vi "Autonomous Independent.vi"() -> ()   [LabVIEW 2020]
doc: "This VI is called when autonomous begins, and will automatically be terminated when autonomous ends. You can carry out timed or sensor driven robot movement independently without needing to return to the caller."
uses:
  <vilib>/Rock Robotics/WPI/DriverStation/WPI_DriverStationAllianceInfo.ctl
  <vilib>/Rock Robotics/Network Tables/NT Read String.vi
  Robot Global Data.vi
panel:
  out "Alliance":T1
  out "Front Left Drive Position":dbl
  out "Navx  Comp Yaw":dbl
  out "Auto Step":dbl
  # "Be sure to right-click and choose Data Operations>>Make Current Value default if you want to save the array values with the VI"
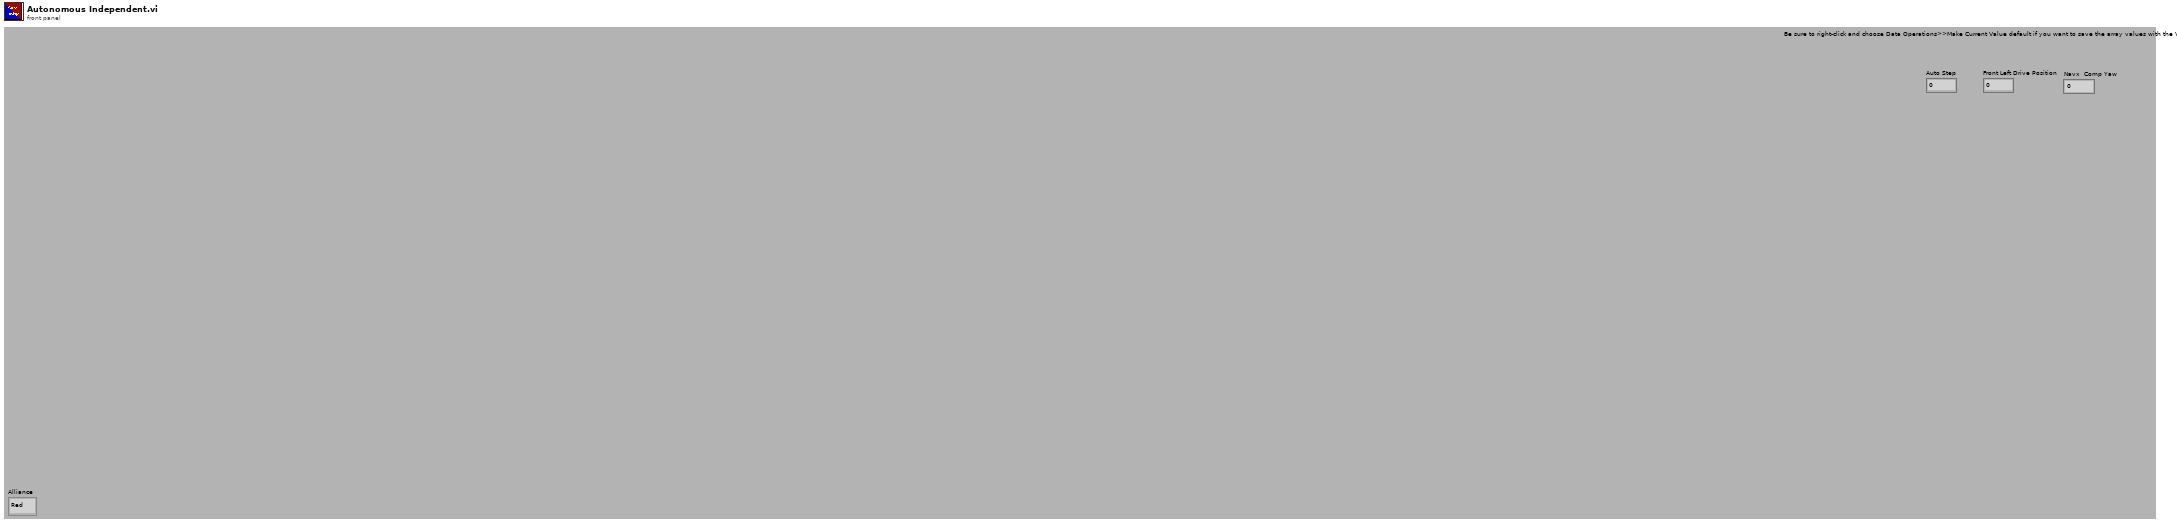
[diagram p1: front panel]
types:
  T1 = typedef "WPI_DriverStationAllianceInfo.ctl" = enum16{"Red", "Blue", "Invalid"}
  T2 = typedef "Direction Commands.ctl" = cluster{"Lateral - X":dbl, "Longitudinal - Y":dbl, "Rotational - Z":dbl}
  T3 = typedef "Drive Comands.ctl" = cluster{"Align Steer Motors":bool, "Brake":bool, "Coast":bool, "Autonomous":bool}
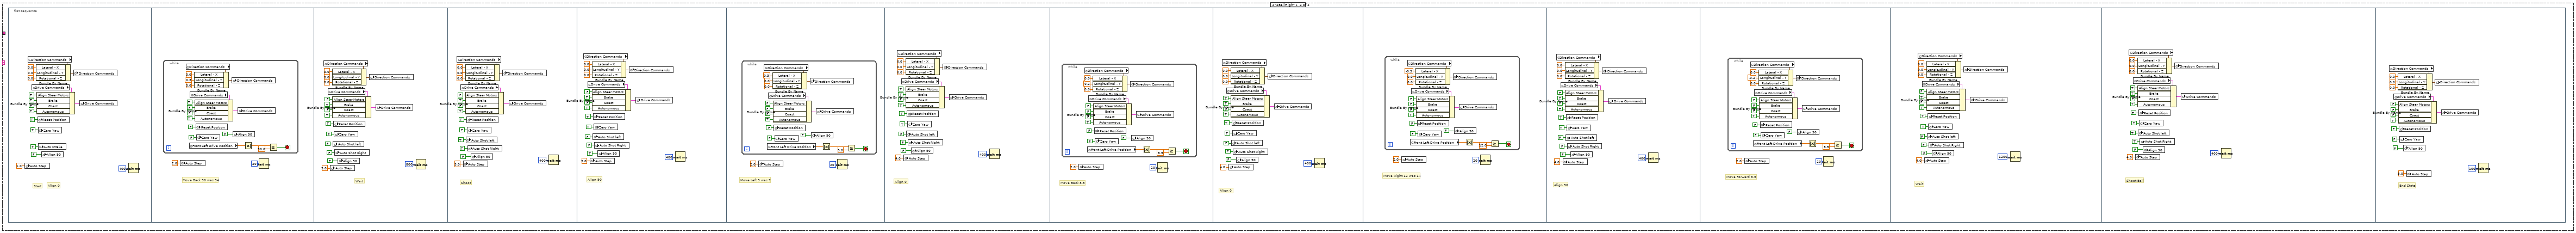
[diagram p2: hidden frame]
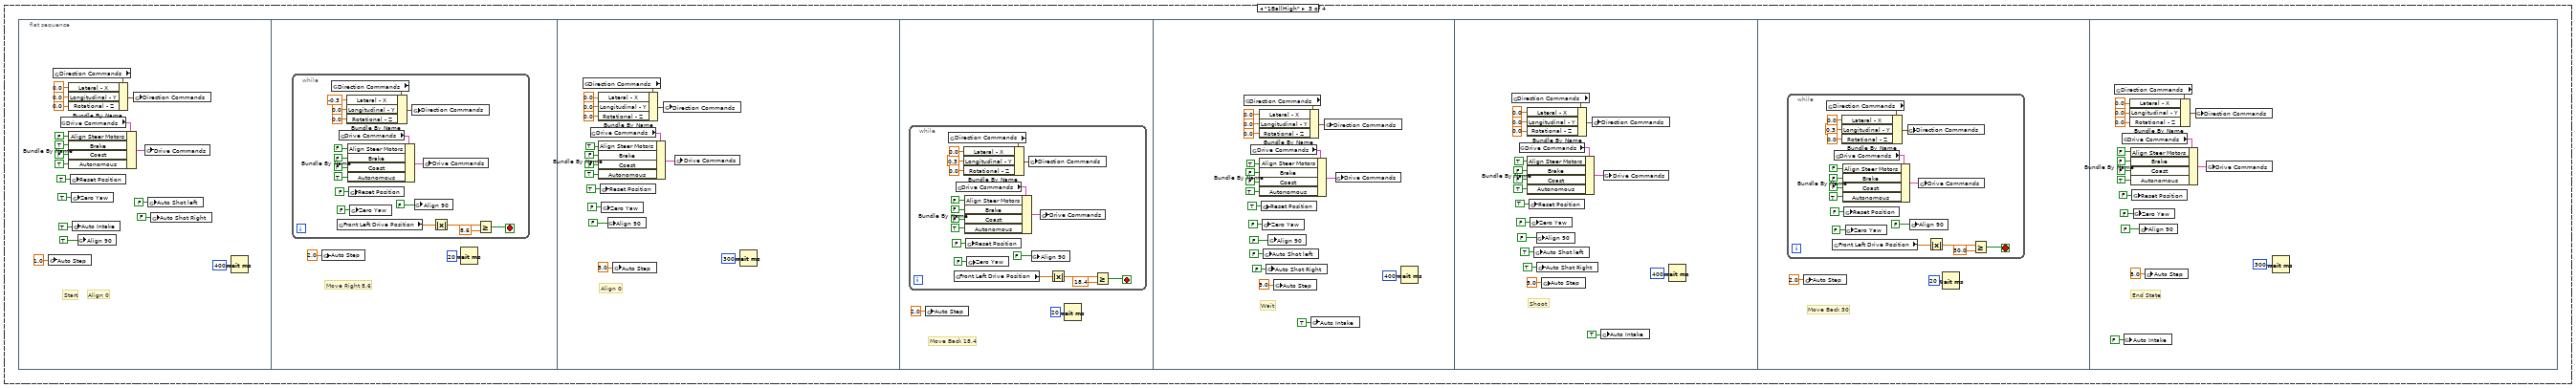
[diagram p3: hidden frame]
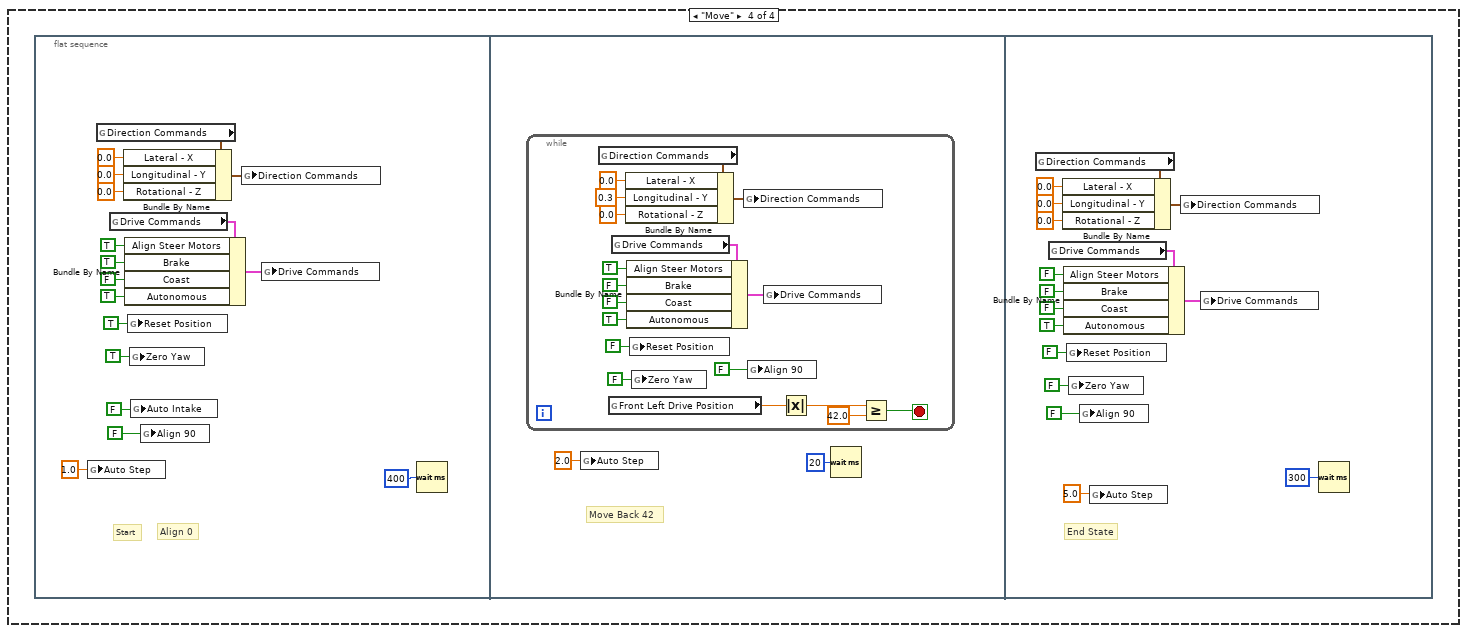
[diagram p4: hidden frame]
diagram:
  (unwired) "This function is run in parallel when the autonomous period begins. It will be terminated automatically when the period ends.\n\nNote that all Driver Station inputs are automatically latched and will not change once auto begins."
  # "Back Long + value\nForward Long - Value\nRight  - Value\nLeft + Value"
  # "The game specific data sent by FMS"
  # "This tells you the autonomous selected in the \ndashboard. Begin.vi publishes the Auto List values\nby writing a constant to the dashboard.\nUpdate the constant to add or modify the name\nof an autonomous."
  # "Every 20ms, report that we are running autonomous\ncode. Loop will abort the same time as the VI."
  # "This tells you the driver position\nand alliance color"
  n1 = call <vilib>:"WPI_DriverStationGet Alliance Info.vi"() -> ("Alliance"=w6:T1)  [unwired: 6 in, 5 out]
  "Alliance" <- w6
  n2 = call <vilib>:"WPI_DriverStationGame Specific Data.vi"() -> ("Game Specific Data"=w7:string)  [unwired: 11 in]
  n3 = while {
    stop <- FALSE stop-if-true
    n4 = call <vilib>:"WPI_DriverStationReport Robot Code State.vi"("Autonomous"=TRUE) -> ()  [unwired: 10 in, 1 out]
    n5 = Wait (ms)(milliseconds to wait=u32 20) -> ()  [unwired: 1 out]
  }
  n6 = Equal?(x=w6, y=WPI_DriverStationAllianceInfo."Red") -> (x = y?=w4:bool)
  n7 = call-poly <vilib>:"NT Read Value.vi"("Name"="Auto Selector") -> ("String"=w8:string)  [unwired: 9 in, 1 out]
  n8 = Select(t="Red" ("Right Color Match 2"), s=w4, f="Blue" ("Right Color Match 2")) -> (s? t:f=w1:string)
  n9 = global write "Robot Global Data.vi" "Alliance Color"(w1) -> ()
  n10 = case shown="\"3Ball\", Default" w8 {
    tunnel: w7 -> [_ _ _ _]
    frame "3Ball", Default {
      n11 = flat-sequence {
        frame #0 {
          # "Align 0"
          # "Start"
          n12 = global write "Robot Global Data.vi" "Auto Step"(1.0 ("Auto Step")) -> ()
          n13 = global read "Robot Global Data.vi" "Direction Commands"() -> (w23:T2)
          n14 = global read "Robot Global Data.vi" "Drive Commands"() -> (w22:T3)
          n15 = Bundle By Name(cluster=w23, "Lateral - X"=0.0, "Longitudinal - Y"=0.0, "Rotational - Z"=0.0) -> (w29:T2)
          n16 = Bundle By Name(cluster=w22, "Align Steer Motors"=TRUE, "Brake"=TRUE, "Coast"=FALSE, "Autonomous"=TRUE) -> (w21:T3)
          n17 = global write "Robot Global Data.vi" "Reset Position"(TRUE ("Reset Position")) -> ()
          n18 = global write "Robot Global Data.vi" "Zero Yaw"(TRUE ("Zero Yaw")) -> ()
          n19 = global write "Robot Global Data.vi" "Auto Intake"(TRUE ("Auto Intake")) -> ()
          n20 = global write "Robot Global Data.vi" "Align 90"(FALSE ("Auto Intake")) -> ()
          n21 = global write "Robot Global Data.vi" "Direction Commands"(w29) -> ()
          n22 = global write "Robot Global Data.vi" "Drive Commands"(w21) -> ()
          n23 = Wait (ms)(milliseconds to wait=u32 400) -> ()  [unwired: 1 out]
        }
        frame #1 {
          # "Move Back 32"
          n24 = while {
            stop <- w34 stop-if-true
            n25 = global read "Robot Global Data.vi" "Direction Commands"() -> (w43:T2)
            n26 = global read "Robot Global Data.vi" "Front Left Drive Position"() -> (w36:dbl)
            n27 = global read "Robot Global Data.vi" "Drive Commands"() -> (w42:T3)
            n28 = Bundle By Name(cluster=w43, "Lateral - X"=0.0, "Longitudinal - Y"=0.3, "Rotational - Z"=0.0) -> (w49:T2)
            n29 = Bundle By Name(cluster=w42, "Align Steer Motors"=TRUE, "Brake"=FALSE, "Coast"=FALSE, "Autonomous"=TRUE) -> (w41:T3)
            n30 = global write "Robot Global Data.vi" "Reset Position"(FALSE ("Reset Position")) -> ()
            n31 = global write "Robot Global Data.vi" "Zero Yaw"(FALSE ("Zero Yaw")) -> ()
            n32 = global write "Robot Global Data.vi" "Direction Commands"(w49) -> ()
            n33 = global write "Robot Global Data.vi" "Align 90"(FALSE ("Auto Intake")) -> ()
            n34 = global write "Robot Global Data.vi" "Drive Commands"(w41) -> ()
            n35 = Absolute Value(x=w36) -> (abs(x)=w33:dbl)
            n36 = Greater Or Equal?(x=w33, y=32.0) -> (x >= y?=w34:bool)
          }
          n37 = global write "Robot Global Data.vi" "Auto Step"(2.0 ("Auto Step")) -> ()
          n38 = Wait (ms)(milliseconds to wait=u32 20) -> ()  [unwired: 1 out]
        }
        frame #2 {
          # "Align 90 Stop"
          n39 = global read "Robot Global Data.vi" "Direction Commands"() -> (w61:T2)
          n40 = global read "Robot Global Data.vi" "Drive Commands"() -> (w60:T3)
          n41 = global write "Robot Global Data.vi" "Auto Step"(3.0 ("Auto Step")) -> ()
          n42 = Bundle By Name(cluster=w61, "Lateral - X"=0.0, "Longitudinal - Y"=0.0, "Rotational - Z"=0.0) -> (w67:T2)
          n43 = Bundle By Name(cluster=w60, "Align Steer Motors"=TRUE, "Brake"=TRUE, "Coast"=FALSE, "Autonomous"=TRUE) -> (w59:T3)
          n44 = global write "Robot Global Data.vi" "Auto Shot left"(FALSE ("Auto Shot left")) -> ()
          n45 = global write "Robot Global Data.vi" "Reset Position"(TRUE ("Reset Position")) -> ()
          n46 = global write "Robot Global Data.vi" "Zero Yaw"(TRUE ("Zero Yaw")) -> ()
          n47 = global write "Robot Global Data.vi" "Auto Shot Right"(FALSE ("Auto Shot Right")) -> ()
          n48 = global write "Robot Global Data.vi" "Align 90"(TRUE ("Auto Intake")) -> ()
          n49 = global write "Robot Global Data.vi" "Direction Commands"(w67) -> ()
          n50 = global write "Robot Global Data.vi" "Drive Commands"(w59) -> ()
          n51 = Wait (ms)(milliseconds to wait=u32 400) -> ()  [unwired: 1 out]
        }
        frame #3 {
          # "Shoot"
          n52 = global read "Robot Global Data.vi" "Direction Commands"() -> (w79:T2)
          n53 = global read "Robot Global Data.vi" "Drive Commands"() -> (w78:T3)
          n54 = global write "Robot Global Data.vi" "Auto Step"(3.0 ("Auto Step")) -> ()
          n55 = Bundle By Name(cluster=w79, "Lateral - X"=0.0, "Longitudinal - Y"=0.0, "Rotational - Z"=0.0) -> (w85:T2)
          n56 = Bundle By Name(cluster=w78, "Align Steer Motors"=TRUE, "Brake"=TRUE, "Coast"=FALSE, "Autonomous"=TRUE) -> (w77:T3)
          n57 = global write "Robot Global Data.vi" "Auto Shot left"(TRUE ("Auto Shot left")) -> ()
          n58 = global write "Robot Global Data.vi" "Reset Position"(TRUE ("Reset Position")) -> ()
          n59 = global write "Robot Global Data.vi" "Zero Yaw"(TRUE ("Zero Yaw")) -> ()
          n60 = global write "Robot Global Data.vi" "Auto Shot Right"(TRUE ("Auto Shot Right")) -> ()
          n61 = global write "Robot Global Data.vi" "Align 90"(TRUE ("Auto Intake")) -> ()
          n62 = global write "Robot Global Data.vi" "Direction Commands"(w85) -> ()
          n63 = global write "Robot Global Data.vi" "Drive Commands"(w77) -> ()
          n64 = Wait (ms)(milliseconds to wait=u32 400) -> ()  [unwired: 1 out]
        }
        frame #4 {
          # "Move Right 6"
          n65 = while {
            stop <- w90 stop-if-true
            n66 = global read "Robot Global Data.vi" "Direction Commands"() -> (w99:T2)
            n67 = global read "Robot Global Data.vi" "Front Left Drive Position"() -> (w92:dbl)
            n68 = global read "Robot Global Data.vi" "Drive Commands"() -> (w98:T3)
            n69 = Bundle By Name(cluster=w99, "Lateral - X"=-0.2, "Longitudinal - Y"=0.0, "Rotational - Z"=0.0) -> (w105:T2)
            n70 = Bundle By Name(cluster=w98, "Align Steer Motors"=FALSE, "Brake"=FALSE, "Coast"=FALSE, "Autonomous"=TRUE) -> (w97:T3)
            n71 = global write "Robot Global Data.vi" "Reset Position"(FALSE ("Reset Position")) -> ()
            n72 = global write "Robot Global Data.vi" "Zero Yaw"(FALSE ("Zero Yaw")) -> ()
            n73 = global write "Robot Global Data.vi" "Direction Commands"(w105) -> ()
            n74 = global write "Robot Global Data.vi" "Align 90"(FALSE ("Auto Intake")) -> ()
            n75 = global write "Robot Global Data.vi" "Drive Commands"(w97) -> ()
            n76 = Absolute Value(x=w92) -> (abs(x)=w89:dbl)
            n77 = Greater Or Equal?(x=w89, y=6.0) -> (x >= y?=w90:bool)
          }
          n78 = global write "Robot Global Data.vi" "Auto Step"(2.0 ("Auto Step")) -> ()
          n79 = Wait (ms)(milliseconds to wait=u32 20) -> ()  [unwired: 1 out]
        }
        frame #5 {
          # "Align 0"
          n80 = global read "Robot Global Data.vi" "Direction Commands"() -> (w117:T2)
          n81 = global read "Robot Global Data.vi" "Drive Commands"() -> (w116:T3)
          n82 = global write "Robot Global Data.vi" "Auto Step"(3.0 ("Auto Step")) -> ()
          n83 = Bundle By Name(cluster=w117, "Lateral - X"=0.0, "Longitudinal - Y"=0.0, "Rotational - Z"=0.0) -> (w123:T2)
          n84 = Bundle By Name(cluster=w116, "Align Steer Motors"=TRUE, "Brake"=TRUE, "Coast"=FALSE, "Autonomous"=TRUE) -> (w115:T3)
          n85 = global write "Robot Global Data.vi" "Auto Shot left"(FALSE ("Auto Shot left")) -> ()
          n86 = global write "Robot Global Data.vi" "Reset Position"(TRUE ("Reset Position")) -> ()
          n87 = global write "Robot Global Data.vi" "Zero Yaw"(TRUE ("Zero Yaw")) -> ()
          n88 = global write "Robot Global Data.vi" "Auto Shot Right"(FALSE ("Auto Shot Right")) -> ()
          n89 = global write "Robot Global Data.vi" "Align 90"(FALSE ("Auto Intake")) -> ()
          n90 = global write "Robot Global Data.vi" "Direction Commands"(w123) -> ()
          n91 = global write "Robot Global Data.vi" "Drive Commands"(w115) -> ()
          n92 = Wait (ms)(milliseconds to wait=u32 400) -> ()  [unwired: 1 out]
        }
        frame #6 {
          # "Move Back 9 was 12"
          n93 = while {
            stop <- w128 stop-if-true
            n94 = global read "Robot Global Data.vi" "Direction Commands"() -> (w137:T2)
            n95 = global read "Robot Global Data.vi" "Front Left Drive Position"() -> (w130:dbl)
            n96 = global read "Robot Global Data.vi" "Drive Commands"() -> (w136:T3)
            n97 = Bundle By Name(cluster=w137, "Lateral - X"=0.0, "Longitudinal - Y"=0.2, "Rotational - Z"=0.0) -> (w143:T2)
            n98 = Bundle By Name(cluster=w136, "Align Steer Motors"=FALSE, "Brake"=FALSE, "Coast"=FALSE, "Autonomous"=TRUE) -> (w135:T3)
            n99 = global write "Robot Global Data.vi" "Reset Position"(FALSE ("Reset Position")) -> ()
            n100 = global write "Robot Global Data.vi" "Zero Yaw"(FALSE ("Zero Yaw")) -> ()
            n101 = global write "Robot Global Data.vi" "Direction Commands"(w143) -> ()
            n102 = global write "Robot Global Data.vi" "Align 90"(FALSE ("Auto Intake")) -> ()
            n103 = global write "Robot Global Data.vi" "Drive Commands"(w135) -> ()
            n104 = Absolute Value(x=w130) -> (abs(x)=w127:dbl)
            n105 = Greater Or Equal?(x=w127, y=9.0) -> (x >= y?=w128:bool)
          }
          n106 = global write "Robot Global Data.vi" "Auto Step"(4.0 ("Auto Step")) -> ()
          n107 = Wait (ms)(milliseconds to wait=u32 20) -> ()  [unwired: 1 out]
        }
        frame #7 {
          # "Align 0"
          n108 = global read "Robot Global Data.vi" "Direction Commands"() -> (w155:T2)
          n109 = global read "Robot Global Data.vi" "Drive Commands"() -> (w154:T3)
          n110 = global write "Robot Global Data.vi" "Auto Step"(5.0 ("Auto Step")) -> ()
          n111 = Bundle By Name(cluster=w155, "Lateral - X"=0.0, "Longitudinal - Y"=0.0, "Rotational - Z"=0.0) -> (w161:T2)
          n112 = Bundle By Name(cluster=w154, "Align Steer Motors"=TRUE, "Brake"=TRUE, "Coast"=FALSE, "Autonomous"=TRUE) -> (w153:T3)
          n113 = global write "Robot Global Data.vi" "Auto Shot left"(FALSE ("Auto Shot left")) -> ()
          n114 = global write "Robot Global Data.vi" "Reset Position"(TRUE ("Reset Position")) -> ()
          n115 = global write "Robot Global Data.vi" "Zero Yaw"(TRUE ("Zero Yaw")) -> ()
          n116 = global write "Robot Global Data.vi" "Auto Shot Right"(FALSE ("Auto Shot Right")) -> ()
          n117 = global write "Robot Global Data.vi" "Direction Commands"(w161) -> ()
          n118 = global write "Robot Global Data.vi" "Drive Commands"(w153) -> ()
          n119 = global write "Robot Global Data.vi" "Align 90"(FALSE ("Auto Intake")) -> ()
          n120 = Wait (ms)(milliseconds to wait=u32 400) -> ()  [unwired: 1 out]
        }
        frame #8 {
          # "Move Forward 30 was 32"
          n121 = while {
            stop <- w166 stop-if-true
            n122 = global read "Robot Global Data.vi" "Direction Commands"() -> (w175:T2)
            n123 = global read "Robot Global Data.vi" "Front Left Drive Position"() -> (w168:dbl)
            n124 = global read "Robot Global Data.vi" "Drive Commands"() -> (w174:T3)
            n125 = Bundle By Name(cluster=w175, "Lateral - X"=0.0, "Longitudinal - Y"=-0.3, "Rotational - Z"=0.0) -> (w181:T2)
            n126 = Bundle By Name(cluster=w174, "Align Steer Motors"=FALSE, "Brake"=FALSE, "Coast"=FALSE, "Autonomous"=TRUE) -> (w173:T3)
            n127 = global write "Robot Global Data.vi" "Reset Position"(FALSE ("Reset Position")) -> ()
            n128 = global write "Robot Global Data.vi" "Zero Yaw"(FALSE ("Zero Yaw")) -> ()
            n129 = global write "Robot Global Data.vi" "Direction Commands"(w181) -> ()
            n130 = global write "Robot Global Data.vi" "Drive Commands"(w173) -> ()
            n131 = Absolute Value(x=w168) -> (abs(x)=w165:dbl)
            n132 = global write "Robot Global Data.vi" "Align 90"(FALSE ("Auto Intake")) -> ()
            n133 = Greater Or Equal?(x=w165, y=30.0) -> (x >= y?=w166:bool)
          }
          n134 = global write "Robot Global Data.vi" "Auto Step"(6.0 ("Auto Step")) -> ()
          n135 = Wait (ms)(milliseconds to wait=u32 20) -> ()  [unwired: 1 out]
        }
        frame #9 {
          # "Align 90"
          n136 = global read "Robot Global Data.vi" "Direction Commands"() -> (w193:T2)
          n137 = global read "Robot Global Data.vi" "Drive Commands"() -> (w192:T3)
          n138 = Bundle By Name(cluster=w193, "Lateral - X"=0.0, "Longitudinal - Y"=0.0, "Rotational - Z"=0.0) -> (w199:T2)
          n139 = Bundle By Name(cluster=w192, "Align Steer Motors"=FALSE, "Brake"=TRUE, "Coast"=FALSE, "Autonomous"=TRUE) -> (w191:T3)
          n140 = global write "Robot Global Data.vi" "Reset Position"(TRUE ("Reset Position")) -> ()
          n141 = global write "Robot Global Data.vi" "Auto Shot left"(FALSE ("Auto Shot left")) -> ()
          n142 = global write "Robot Global Data.vi" "Zero Yaw"(TRUE ("Zero Yaw")) -> ()
          n143 = global write "Robot Global Data.vi" "Auto Shot Right"(FALSE ("Auto Shot Right")) -> ()
          n144 = global write "Robot Global Data.vi" "Auto Step"(7.0 ("Auto Step")) -> ()
          n145 = global write "Robot Global Data.vi" "Direction Commands"(w199) -> ()
          n146 = global write "Robot Global Data.vi" "Drive Commands"(w191) -> ()
          n147 = global write "Robot Global Data.vi" "Align 90"(TRUE ("Auto Intake")) -> ()
          n148 = Wait (ms)(milliseconds to wait=u32 400) -> ()  [unwired: 1 out]
        }
        frame #10 {
          # "Move Left 57 was 51"
          n149 = while {
            stop <- w204 stop-if-true
            n150 = global read "Robot Global Data.vi" "Direction Commands"() -> (w213:T2)
            n151 = global read "Robot Global Data.vi" "Front Left Drive Position"() -> (w206:dbl)
            n152 = global read "Robot Global Data.vi" "Drive Commands"() -> (w212:T3)
            n153 = Bundle By Name(cluster=w213, "Lateral - X"=0.3, "Longitudinal - Y"=0.0, "Rotational - Z"=0.0) -> (w219:T2)
            n154 = Bundle By Name(cluster=w212, "Align Steer Motors"=FALSE, "Brake"=FALSE, "Coast"=FALSE, "Autonomous"=TRUE) -> (w211:T3)
            n155 = global write "Robot Global Data.vi" "Reset Position"(FALSE ("Reset Position")) -> ()
            n156 = global write "Robot Global Data.vi" "Zero Yaw"(FALSE ("Zero Yaw")) -> ()
            n157 = global write "Robot Global Data.vi" "Direction Commands"(w219) -> ()
            n158 = global write "Robot Global Data.vi" "Drive Commands"(w211) -> ()
            n159 = Absolute Value(x=w206) -> (abs(x)=w203:dbl)
            n160 = global write "Robot Global Data.vi" "Align 90"(FALSE ("Auto Intake")) -> ()
            n161 = Greater Or Equal?(x=w203, y=57.0) -> (x >= y?=w204:bool)
          }
          n162 = global write "Robot Global Data.vi" "Auto Step"(8.0 ("Auto Step")) -> ()
          n163 = Wait (ms)(milliseconds to wait=u32 20) -> ()  [unwired: 1 out]
        }
        frame #11 {
          # "Aign 0"
          n164 = global read "Robot Global Data.vi" "Direction Commands"() -> (w231:T2)
          n165 = global read "Robot Global Data.vi" "Drive Commands"() -> (w230:T3)
          n166 = global write "Robot Global Data.vi" "Auto Step"(5.0 ("Auto Step")) -> ()
          n167 = Bundle By Name(cluster=w231, "Lateral - X"=0.0, "Longitudinal - Y"=0.0, "Rotational - Z"=0.0) -> (w237:T2)
          n168 = Bundle By Name(cluster=w230, "Align Steer Motors"=TRUE, "Brake"=TRUE, "Coast"=FALSE, "Autonomous"=TRUE) -> (w229:T3)
          n169 = global write "Robot Global Data.vi" "Auto Shot left"(FALSE ("Auto Shot left")) -> ()
          n170 = global write "Robot Global Data.vi" "Reset Position"(TRUE ("Reset Position")) -> ()
          n171 = global write "Robot Global Data.vi" "Zero Yaw"(TRUE ("Zero Yaw")) -> ()
          n172 = global write "Robot Global Data.vi" "Auto Shot Right"(FALSE ("Auto Shot Right")) -> ()
          n173 = global write "Robot Global Data.vi" "Direction Commands"(w237) -> ()
          n174 = global write "Robot Global Data.vi" "Drive Commands"(w229) -> ()
          n175 = global write "Robot Global Data.vi" "Align 90"(FALSE ("Auto Intake")) -> ()
          n176 = Wait (ms)(milliseconds to wait=u32 400) -> ()  [unwired: 1 out]
        }
        frame #12 {
          # "Move Back 12 was 19"
          n177 = while {
            stop <- w242 stop-if-true
            n178 = global read "Robot Global Data.vi" "Direction Commands"() -> (w251:T2)
            n179 = global read "Robot Global Data.vi" "Front Left Drive Position"() -> (w244:dbl)
            n180 = global read "Robot Global Data.vi" "Drive Commands"() -> (w250:T3)
            n181 = Bundle By Name(cluster=w251, "Lateral - X"=0.0, "Longitudinal - Y"=0.3, "Rotational - Z"=0.0) -> (w257:T2)
            n182 = Bundle By Name(cluster=w250, "Align Steer Motors"=FALSE, "Brake"=FALSE, "Coast"=FALSE, "Autonomous"=TRUE) -> (w249:T3)
            n183 = global write "Robot Global Data.vi" "Reset Position"(FALSE ("Reset Position")) -> ()
            n184 = global write "Robot Global Data.vi" "Zero Yaw"(FALSE ("Zero Yaw")) -> ()
            n185 = global write "Robot Global Data.vi" "Direction Commands"(w257) -> ()
            n186 = global write "Robot Global Data.vi" "Drive Commands"(w249) -> ()
            n187 = Absolute Value(x=w244) -> (abs(x)=w241:dbl)
            n188 = global write "Robot Global Data.vi" "Align 90"(FALSE ("Auto Intake")) -> ()
            n189 = Greater Or Equal?(x=w241, y=12.0) -> (x >= y?=w242:bool)
          }
          n190 = global write "Robot Global Data.vi" "Auto Step"(6.0 ("Auto Step")) -> ()
          n191 = Wait (ms)(milliseconds to wait=u32 20) -> ()  [unwired: 1 out]
        }
        frame #13 {
          # "Align 90"
          n192 = global read "Robot Global Data.vi" "Direction Commands"() -> (w269:T2)
          n193 = global read "Robot Global Data.vi" "Drive Commands"() -> (w268:T3)
          n194 = Bundle By Name(cluster=w269, "Lateral - X"=0.0, "Longitudinal - Y"=0.0, "Rotational - Z"=0.0) -> (w275:T2)
          n195 = Bundle By Name(cluster=w268, "Align Steer Motors"=FALSE, "Brake"=TRUE, "Coast"=FALSE, "Autonomous"=TRUE) -> (w267:T3)
          n196 = global write "Robot Global Data.vi" "Reset Position"(TRUE ("Reset Position")) -> ()
          n197 = global write "Robot Global Data.vi" "Auto Shot left"(FALSE ("Auto Shot left")) -> ()
          n198 = global write "Robot Global Data.vi" "Zero Yaw"(TRUE ("Zero Yaw")) -> ()
          n199 = global write "Robot Global Data.vi" "Auto Shot Right"(FALSE ("Auto Shot Right")) -> ()
          n200 = global write "Robot Global Data.vi" "Auto Step"(7.0 ("Auto Step")) -> ()
          n201 = global write "Robot Global Data.vi" "Direction Commands"(w275) -> ()
          n202 = global write "Robot Global Data.vi" "Drive Commands"(w267) -> ()
          n203 = global write "Robot Global Data.vi" "Align 90"(TRUE ("Auto Intake")) -> ()
          n204 = Wait (ms)(milliseconds to wait=u32 400) -> ()  [unwired: 1 out]
        }
        frame #14 {
          # "Move Right  45 was 48 was 39"
          n205 = while {
            stop <- w280 stop-if-true
            n206 = global read "Robot Global Data.vi" "Direction Commands"() -> (w289:T2)
            n207 = global read "Robot Global Data.vi" "Front Left Drive Position"() -> (w282:dbl)
            n208 = global read "Robot Global Data.vi" "Drive Commands"() -> (w288:T3)
            n209 = Bundle By Name(cluster=w289, "Lateral - X"=-0.3, "Longitudinal - Y"=0.0, "Rotational - Z"=0.0) -> (w295:T2)
            n210 = Bundle By Name(cluster=w288, "Align Steer Motors"=FALSE, "Brake"=FALSE, "Coast"=FALSE, "Autonomous"=TRUE) -> (w287:T3)
            n211 = global write "Robot Global Data.vi" "Reset Position"(FALSE ("Reset Position")) -> ()
            n212 = global write "Robot Global Data.vi" "Zero Yaw"(FALSE ("Zero Yaw")) -> ()
            n213 = global write "Robot Global Data.vi" "Direction Commands"(w295) -> ()
            n214 = global write "Robot Global Data.vi" "Drive Commands"(w287) -> ()
            n215 = Absolute Value(x=w282) -> (abs(x)=w279:dbl)
            n216 = global write "Robot Global Data.vi" "Align 90"(FALSE ("Auto Intake")) -> ()
            n217 = Greater Or Equal?(x=w279, y=45.0) -> (x >= y?=w280:bool)
          }
          n218 = global write "Robot Global Data.vi" "Auto Step"(8.0 ("Auto Step")) -> ()
          n219 = Wait (ms)(milliseconds to wait=u32 20) -> ()  [unwired: 1 out]
        }
        frame #15 {
          # "Align 0"
          n220 = global read "Robot Global Data.vi" "Direction Commands"() -> (w305:T2)
          n221 = global read "Robot Global Data.vi" "Drive Commands"() -> (w306:T3)
          n222 = global write "Robot Global Data.vi" "Auto Shot left"(FALSE ("Auto Shot left")) -> ()
          n223 = global write "Robot Global Data.vi" "Auto Shot Right"(FALSE ("Auto Shot Right")) -> ()
          n224 = Bundle By Name(cluster=w305, "Lateral - X"=0.0, "Longitudinal - Y"=0.0, "Rotational - Z"=0.0) -> (w299:T2)
          n225 = Bundle By Name(cluster=w306, "Align Steer Motors"=TRUE, "Brake"=TRUE, "Coast"=FALSE, "Autonomous"=TRUE) -> (w307:T3)
          n226 = global write "Robot Global Data.vi" "Reset Position"(TRUE ("Reset Position")) -> ()
          n227 = global write "Robot Global Data.vi" "Zero Yaw"(TRUE ("Zero Yaw")) -> ()
          n228 = global write "Robot Global Data.vi" "Auto Step"(9.0 ("Auto Step")) -> ()
          n229 = global write "Robot Global Data.vi" "Direction Commands"(w299) -> ()
          n230 = global write "Robot Global Data.vi" "Drive Commands"(w307) -> ()
          n231 = global write "Robot Global Data.vi" "Align 90"(FALSE ("Auto Intake")) -> ()
          n232 = Wait (ms)(milliseconds to wait=u32 400) -> ()  [unwired: 1 out]
        }
        frame #16 {
          # "Wait"
          n233 = global read "Robot Global Data.vi" "Direction Commands"() -> (w325:T2)
          n234 = global read "Robot Global Data.vi" "Drive Commands"() -> (w324:T3)
          n235 = global write "Robot Global Data.vi" "Auto Step"(4.0 ("Auto Step")) -> ()
          n236 = Bundle By Name(cluster=w325, "Lateral - X"=0.0, "Longitudinal - Y"=0.0, "Rotational - Z"=0.0) -> (w331:T2)
          n237 = Bundle By Name(cluster=w324, "Align Steer Motors"=FALSE, "Brake"=TRUE, "Coast"=FALSE, "Autonomous"=TRUE) -> (w323:T3)
          n238 = global write "Robot Global Data.vi" "Auto Shot left"(FALSE ("Auto Shot left")) -> ()
          n239 = global write "Robot Global Data.vi" "Reset Position"(TRUE ("Reset Position")) -> ()
          n240 = global write "Robot Global Data.vi" "Zero Yaw"(TRUE ("Zero Yaw")) -> ()
          n241 = global write "Robot Global Data.vi" "Auto Shot Right"(FALSE ("Auto Shot Right")) -> ()
          n242 = global write "Robot Global Data.vi" "Align 90"(FALSE ("Auto Intake")) -> ()
          n243 = global write "Robot Global Data.vi" "Direction Commands"(w331) -> ()
          n244 = global write "Robot Global Data.vi" "Drive Commands"(w323) -> ()
          n245 = Wait (ms)(milliseconds to wait=u32 800) -> ()  [unwired: 1 out]
        }
        frame #17 {
          # "Align 0"
          n246 = global read "Robot Global Data.vi" "Direction Commands"() -> (w341:T2)
          n247 = global read "Robot Global Data.vi" "Drive Commands"() -> (w342:T3)
          n248 = global write "Robot Global Data.vi" "Auto Shot left"(FALSE ("Auto Shot left")) -> ()
          n249 = global write "Robot Global Data.vi" "Auto Shot Right"(FALSE ("Auto Shot Right")) -> ()
          n250 = Bundle By Name(cluster=w341, "Lateral - X"=0.0, "Longitudinal - Y"=0.0, "Rotational - Z"=0.0) -> (w335:T2)
          n251 = Bundle By Name(cluster=w342, "Align Steer Motors"=TRUE, "Brake"=TRUE, "Coast"=FALSE, "Autonomous"=TRUE) -> (w343:T3)
          n252 = global write "Robot Global Data.vi" "Reset Position"(TRUE ("Reset Position")) -> ()
          n253 = global write "Robot Global Data.vi" "Zero Yaw"(TRUE ("Zero Yaw")) -> ()
          n254 = global write "Robot Global Data.vi" "Auto Step"(9.0 ("Auto Step")) -> ()
          n255 = global write "Robot Global Data.vi" "Direction Commands"(w335) -> ()
          n256 = global write "Robot Global Data.vi" "Drive Commands"(w343) -> ()
          n257 = global write "Robot Global Data.vi" "Align 90"(FALSE ("Auto Intake")) -> ()
          n258 = Wait (ms)(milliseconds to wait=u32 400) -> ()  [unwired: 1 out]
        }
        frame #18 {
          # "Align 0 and Shoot"
          n259 = global read "Robot Global Data.vi" "Direction Commands"() -> (w359:T2)
          n260 = global read "Robot Global Data.vi" "Drive Commands"() -> (w360:T3)
          n261 = Bundle By Name(cluster=w359, "Lateral - X"=0.0, "Longitudinal - Y"=0.0, "Rotational - Z"=0.0) -> (w353:T2)
          n262 = Bundle By Name(cluster=w360, "Align Steer Motors"=TRUE, "Brake"=TRUE, "Coast"=FALSE, "Autonomous"=TRUE) -> (w361:T3)
          n263 = global write "Robot Global Data.vi" "Reset Position"(TRUE ("Reset Position")) -> ()
          n264 = global write "Robot Global Data.vi" "Zero Yaw"(TRUE ("Zero Yaw")) -> ()
          n265 = global write "Robot Global Data.vi" "Align 90"(FALSE ("Auto Intake")) -> ()
          n266 = global write "Robot Global Data.vi" "Auto Step"(11.0 ("Auto Step")) -> ()
          n267 = global write "Robot Global Data.vi" "Direction Commands"(w353) -> ()
          n268 = global write "Robot Global Data.vi" "Drive Commands"(w361) -> ()
          n269 = global write "Robot Global Data.vi" "Auto Shot left"(TRUE ("Auto Shot left")) -> ()
          n270 = global write "Robot Global Data.vi" "Auto Shot Right"(FALSE ("Auto Shot Right")) -> ()
          n271 = Wait (ms)(milliseconds to wait=u32 200) -> ()  [unwired: 1 out]
        }
        frame #19 {
          # "Align 0 and Shoot"
          n272 = global read "Robot Global Data.vi" "Direction Commands"() -> (w377:T2)
          n273 = global read "Robot Global Data.vi" "Drive Commands"() -> (w378:T3)
          n274 = Bundle By Name(cluster=w377, "Lateral - X"=0.0, "Longitudinal - Y"=0.0, "Rotational - Z"=0.0) -> (w371:T2)
          n275 = Bundle By Name(cluster=w378, "Align Steer Motors"=TRUE, "Brake"=TRUE, "Coast"=FALSE, "Autonomous"=TRUE) -> (w379:T3)
          n276 = global write "Robot Global Data.vi" "Reset Position"(TRUE ("Reset Position")) -> ()
          n277 = global write "Robot Global Data.vi" "Zero Yaw"(TRUE ("Zero Yaw")) -> ()
          n278 = global write "Robot Global Data.vi" "Align 90"(FALSE ("Auto Intake")) -> ()
          n279 = global write "Robot Global Data.vi" "Auto Step"(11.0 ("Auto Step")) -> ()
          n280 = global write "Robot Global Data.vi" "Direction Commands"(w371) -> ()
          n281 = global write "Robot Global Data.vi" "Drive Commands"(w379) -> ()
          n282 = global write "Robot Global Data.vi" "Auto Shot left"(FALSE ("Auto Shot left")) -> ()
          n283 = global write "Robot Global Data.vi" "Auto Shot Right"(TRUE ("Auto Shot Right")) -> ()
          n284 = Wait (ms)(milliseconds to wait=u32 200) -> ()  [unwired: 1 out]
        }
        frame #20 {
          # "End State"
          n285 = global read "Robot Global Data.vi" "Direction Commands"() -> (w395:T2)
          n286 = global read "Robot Global Data.vi" "Drive Commands"() -> (w394:T3)
          n287 = Bundle By Name(cluster=w395, "Lateral - X"=0.0, "Longitudinal - Y"=0.0, "Rotational - Z"=0.0) -> (w401:T2)
          n288 = Bundle By Name(cluster=w394, "Align Steer Motors"=FALSE, "Brake"=FALSE, "Coast"=FALSE, "Autonomous"=TRUE) -> (w393:T3)
          n289 = global write "Robot Global Data.vi" "Reset Position"(FALSE ("Reset Position")) -> ()
          n290 = global write "Robot Global Data.vi" "Zero Yaw"(FALSE ("Zero Yaw")) -> ()
          n291 = global write "Robot Global Data.vi" "Align 90"(FALSE ("Auto Intake")) -> ()
          n292 = global write "Robot Global Data.vi" "Auto Step"(18.0 ("Auto Step")) -> ()
          n293 = global write "Robot Global Data.vi" "Direction Commands"(w401) -> ()
          n294 = global write "Robot Global Data.vi" "Drive Commands"(w393) -> ()
          n295 = Wait (ms)(milliseconds to wait=u32 300) -> ()  [unwired: 1 out]
        }
      }
    }
    frame "2BallHigh" {
      n296 = flat-sequence {
        frame #0 {
          # "Align 0"
          # "Start"
          n297 = global write "Robot Global Data.vi" "Auto Step"(1.0 ("Auto Step")) -> ()
          n298 = global read "Robot Global Data.vi" "Direction Commands"() -> (w412:T2)
          n299 = global read "Robot Global Data.vi" "Drive Commands"() -> (w411:T3)
          n300 = Bundle By Name(cluster=w412, "Lateral - X"=0.0, "Longitudinal - Y"=0.0, "Rotational - Z"=0.0) -> (w418:T2)
          n301 = Bundle By Name(cluster=w411, "Align Steer Motors"=TRUE, "Brake"=TRUE, "Coast"=FALSE, "Autonomous"=TRUE) -> (w410:T3)
          n302 = global write "Robot Global Data.vi" "Reset Position"(TRUE ("Reset Position")) -> ()
          n303 = global write "Robot Global Data.vi" "Zero Yaw"(TRUE ("Zero Yaw")) -> ()
          n304 = global write "Robot Global Data.vi" "Auto Intake"(TRUE ("Auto Intake")) -> ()
          n305 = global write "Robot Global Data.vi" "Align 90"(FALSE ("Auto Intake")) -> ()
          n306 = global write "Robot Global Data.vi" "Direction Commands"(w418) -> ()
          n307 = global write "Robot Global Data.vi" "Drive Commands"(w410) -> ()
          n308 = Wait (ms)(milliseconds to wait=u32 400) -> ()  [unwired: 1 out]
        }
        frame #1 {
          # "Move Back 30 was 34"
          n309 = while {
            stop <- w423 stop-if-true
            n310 = global read "Robot Global Data.vi" "Direction Commands"() -> (w432:T2)
            n311 = global read "Robot Global Data.vi" "Front Left Drive Position"() -> (w425:dbl)
            n312 = global read "Robot Global Data.vi" "Drive Commands"() -> (w431:T3)
            n313 = Bundle By Name(cluster=w432, "Lateral - X"=0.0, "Longitudinal - Y"=0.3, "Rotational - Z"=0.0) -> (w438:T2)
            n314 = Bundle By Name(cluster=w431, "Align Steer Motors"=TRUE, "Brake"=FALSE, "Coast"=FALSE, "Autonomous"=TRUE) -> (w430:T3)
            n315 = global write "Robot Global Data.vi" "Reset Position"(FALSE ("Reset Position")) -> ()
            n316 = global write "Robot Global Data.vi" "Zero Yaw"(FALSE ("Zero Yaw")) -> ()
            n317 = global write "Robot Global Data.vi" "Direction Commands"(w438) -> ()
            n318 = global write "Robot Global Data.vi" "Align 90"(FALSE ("Auto Intake")) -> ()
            n319 = global write "Robot Global Data.vi" "Drive Commands"(w430) -> ()
            n320 = Absolute Value(x=w425) -> (abs(x)=w422:dbl)
            n321 = Greater Or Equal?(x=w422, y=30.0) -> (x >= y?=w423:bool)
          }
          n322 = global write "Robot Global Data.vi" "Auto Step"(2.0 ("Auto Step")) -> ()
          n323 = Wait (ms)(milliseconds to wait=u32 20) -> ()  [unwired: 1 out]
        }
        frame #2 {
          # "Wait"
          n324 = global read "Robot Global Data.vi" "Direction Commands"() -> (w450:T2)
          n325 = global read "Robot Global Data.vi" "Drive Commands"() -> (w449:T3)
          n326 = global write "Robot Global Data.vi" "Auto Step"(3.0 ("Auto Step")) -> ()
          n327 = Bundle By Name(cluster=w450, "Lateral - X"=0.0, "Longitudinal - Y"=0.0, "Rotational - Z"=0.0) -> (w456:T2)
          n328 = Bundle By Name(cluster=w449, "Align Steer Motors"=FALSE, "Brake"=TRUE, "Coast"=FALSE, "Autonomous"=TRUE) -> (w448:T3)
          n329 = global write "Robot Global Data.vi" "Auto Shot left"(FALSE ("Auto Shot left")) -> ()
          n330 = global write "Robot Global Data.vi" "Reset Position"(TRUE ("Reset Position")) -> ()
          n331 = global write "Robot Global Data.vi" "Zero Yaw"(FALSE ("Zero Yaw")) -> ()
          n332 = global write "Robot Global Data.vi" "Auto Shot Right"(FALSE ("Auto Shot Right")) -> ()
          n333 = global write "Robot Global Data.vi" "Align 90"(FALSE ("Auto Intake")) -> ()
          n334 = global write "Robot Global Data.vi" "Direction Commands"(w456) -> ()
          n335 = global write "Robot Global Data.vi" "Drive Commands"(w448) -> ()
          n336 = Wait (ms)(milliseconds to wait=u32 800) -> ()  [unwired: 1 out]
        }
        frame #3 {
          # "Shoot"
          n337 = global read "Robot Global Data.vi" "Direction Commands"() -> (w468:T2)
          n338 = global read "Robot Global Data.vi" "Drive Commands"() -> (w467:T3)
          n339 = global write "Robot Global Data.vi" "Auto Step"(3.0 ("Auto Step")) -> ()
          n340 = Bundle By Name(cluster=w468, "Lateral - X"=0.0, "Longitudinal - Y"=0.0, "Rotational - Z"=0.0) -> (w474:T2)
          n341 = Bundle By Name(cluster=w467, "Align Steer Motors"=FALSE, "Brake"=TRUE, "Coast"=FALSE, "Autonomous"=TRUE) -> (w466:T3)
          n342 = global write "Robot Global Data.vi" "Auto Shot left"(TRUE ("Auto Shot left")) -> ()
          n343 = global write "Robot Global Data.vi" "Reset Position"(TRUE ("Reset Position")) -> ()
          n344 = global write "Robot Global Data.vi" "Zero Yaw"(FALSE ("Zero Yaw")) -> ()
          n345 = global write "Robot Global Data.vi" "Auto Shot Right"(TRUE ("Auto Shot Right")) -> ()
          n346 = global write "Robot Global Data.vi" "Align 90"(FALSE ("Auto Intake")) -> ()
          n347 = global write "Robot Global Data.vi" "Direction Commands"(w474) -> ()
          n348 = global write "Robot Global Data.vi" "Drive Commands"(w466) -> ()
          n349 = Wait (ms)(milliseconds to wait=u32 400) -> ()  [unwired: 1 out]
        }
        frame #4 {
          # "Align 90"
          n350 = global read "Robot Global Data.vi" "Direction Commands"() -> (w486:T2)
          n351 = global read "Robot Global Data.vi" "Drive Commands"() -> (w485:T3)
          n352 = global write "Robot Global Data.vi" "Auto Step"(3.0 ("Auto Step")) -> ()
          n353 = Bundle By Name(cluster=w486, "Lateral - X"=0.0, "Longitudinal - Y"=0.0, "Rotational - Z"=0.0) -> (w492:T2)
          n354 = Bundle By Name(cluster=w485, "Align Steer Motors"=FALSE, "Brake"=TRUE, "Coast"=FALSE, "Autonomous"=TRUE) -> (w484:T3)
          n355 = global write "Robot Global Data.vi" "Auto Shot left"(FALSE ("Auto Shot left")) -> ()
          n356 = global write "Robot Global Data.vi" "Reset Position"(TRUE ("Reset Position")) -> ()
          n357 = global write "Robot Global Data.vi" "Zero Yaw"(TRUE ("Zero Yaw")) -> ()
          n358 = global write "Robot Global Data.vi" "Auto Shot Right"(FALSE ("Auto Shot Right")) -> ()
          n359 = global write "Robot Global Data.vi" "Align 90"(TRUE ("Auto Intake")) -> ()
          n360 = global write "Robot Global Data.vi" "Direction Commands"(w492) -> ()
          n361 = global write "Robot Global Data.vi" "Drive Commands"(w484) -> ()
          n362 = Wait (ms)(milliseconds to wait=u32 400) -> ()  [unwired: 1 out]
        }
        frame #5 {
          # "Move Left 5 was 7"
          n363 = while {
            stop <- w497 stop-if-true
            n364 = global read "Robot Global Data.vi" "Direction Commands"() -> (w506:T2)
            n365 = global read "Robot Global Data.vi" "Front Left Drive Position"() -> (w499:dbl)
            n366 = global read "Robot Global Data.vi" "Drive Commands"() -> (w505:T3)
            n367 = Bundle By Name(cluster=w506, "Lateral - X"=0.3, "Longitudinal - Y"=0.0, "Rotational - Z"=0.0) -> (w512:T2)
            n368 = Bundle By Name(cluster=w505, "Align Steer Motors"=FALSE, "Brake"=FALSE, "Coast"=FALSE, "Autonomous"=TRUE) -> (w504:T3)
            n369 = global write "Robot Global Data.vi" "Reset Position"(FALSE ("Reset Position")) -> ()
            n370 = global write "Robot Global Data.vi" "Zero Yaw"(FALSE ("Zero Yaw")) -> ()
            n371 = global write "Robot Global Data.vi" "Direction Commands"(w512) -> ()
            n372 = global write "Robot Global Data.vi" "Align 90"(FALSE ("Auto Intake")) -> ()
            n373 = global write "Robot Global Data.vi" "Drive Commands"(w504) -> ()
            n374 = Absolute Value(x=w499) -> (abs(x)=w496:dbl)
            n375 = Greater Or Equal?(x=w496, y=5.0) -> (x >= y?=w497:bool)
          }
          n376 = global write "Robot Global Data.vi" "Auto Step"(2.0 ("Auto Step")) -> ()
          n377 = Wait (ms)(milliseconds to wait=u32 20) -> ()  [unwired: 1 out]
        }
        frame #6 {
          # "Align 0"
          n378 = global read "Robot Global Data.vi" "Direction Commands"() -> (w524:T2)
          n379 = global read "Robot Global Data.vi" "Drive Commands"() -> (w523:T3)
          n380 = global write "Robot Global Data.vi" "Auto Step"(4.0 ("Auto Step")) -> ()
          n381 = Bundle By Name(cluster=w524, "Lateral - X"=0.0, "Longitudinal - Y"=0.0, "Rotational - Z"=0.0) -> (w530:T2)
          n382 = Bundle By Name(cluster=w523, "Align Steer Motors"=TRUE, "Brake"=TRUE, "Coast"=FALSE, "Autonomous"=TRUE) -> (w522:T3)
          n383 = global write "Robot Global Data.vi" "Auto Shot left"(FALSE ("Auto Shot left")) -> ()
          n384 = global write "Robot Global Data.vi" "Reset Position"(TRUE ("Reset Position")) -> ()
          n385 = global write "Robot Global Data.vi" "Zero Yaw"(TRUE ("Zero Yaw")) -> ()
          n386 = global write "Robot Global Data.vi" "Auto Shot Right"(FALSE ("Auto Shot Right")) -> ()
          n387 = global write "Robot Global Data.vi" "Align 90"(FALSE ("Auto Intake")) -> ()
          n388 = global write "Robot Global Data.vi" "Direction Commands"(w530) -> ()
          n389 = global write "Robot Global Data.vi" "Drive Commands"(w522) -> ()
          n390 = Wait (ms)(milliseconds to wait=u32 400) -> ()  [unwired: 1 out]
        }
        frame #7 {
          # "Move Back 8.5"
          n391 = while {
            stop <- w535 stop-if-true
            n392 = global read "Robot Global Data.vi" "Direction Commands"() -> (w544:T2)
            n393 = global read "Robot Global Data.vi" "Front Left Drive Position"() -> (w537:dbl)
            n394 = global read "Robot Global Data.vi" "Drive Commands"() -> (w543:T3)
            n395 = Bundle By Name(cluster=w544, "Lateral - X"=0.0, "Longitudinal - Y"=0.2, "Rotational - Z"=0.0) -> (w550:T2)
            n396 = Bundle By Name(cluster=w543, "Align Steer Motors"=FALSE, "Brake"=FALSE, "Coast"=FALSE, "Autonomous"=TRUE) -> (w542:T3)
            n397 = global write "Robot Global Data.vi" "Reset Position"(FALSE ("Reset Position")) -> ()
            n398 = global write "Robot Global Data.vi" "Zero Yaw"(FALSE ("Zero Yaw")) -> ()
            n399 = global write "Robot Global Data.vi" "Direction Commands"(w550) -> ()
            n400 = global write "Robot Global Data.vi" "Align 90"(FALSE ("Auto Intake")) -> ()
            n401 = global write "Robot Global Data.vi" "Drive Commands"(w542) -> ()
            n402 = Absolute Value(x=w537) -> (abs(x)=w534:dbl)
            n403 = Greater Or Equal?(x=w534, y=8.5) -> (x >= y?=w535:bool)
          }
          n404 = global write "Robot Global Data.vi" "Auto Step"(2.0 ("Auto Step")) -> ()
          n405 = Wait (ms)(milliseconds to wait=u32 20) -> ()  [unwired: 1 out]
        }
        frame #8 {
          # "Align 0"
          n406 = global read "Robot Global Data.vi" "Direction Commands"() -> (w562:T2)
          n407 = global read "Robot Global Data.vi" "Drive Commands"() -> (w561:T3)
          n408 = global write "Robot Global Data.vi" "Auto Step"(4.0 ("Auto Step")) -> ()
          n409 = Bundle By Name(cluster=w562, "Lateral - X"=0.0, "Longitudinal - Y"=0.0, "Rotational - Z"=0.0) -> (w568:T2)
          n410 = Bundle By Name(cluster=w561, "Align Steer Motors"=TRUE, "Brake"=TRUE, "Coast"=FALSE, "Autonomous"=TRUE) -> (w560:T3)
          n411 = global write "Robot Global Data.vi" "Auto Shot left"(FALSE ("Auto Shot left")) -> ()
          n412 = global write "Robot Global Data.vi" "Reset Position"(TRUE ("Reset Position")) -> ()
          n413 = global write "Robot Global Data.vi" "Zero Yaw"(TRUE ("Zero Yaw")) -> ()
          n414 = global write "Robot Global Data.vi" "Auto Shot Right"(FALSE ("Auto Shot Right")) -> ()
          n415 = global write "Robot Global Data.vi" "Align 90"(FALSE ("Auto Intake")) -> ()
          n416 = global write "Robot Global Data.vi" "Direction Commands"(w568) -> ()
          n417 = global write "Robot Global Data.vi" "Drive Commands"(w560) -> ()
          n418 = Wait (ms)(milliseconds to wait=u32 400) -> ()  [unwired: 1 out]
        }
        frame #9 {
          # "Move Right 12 was 14"
          n419 = while {
            stop <- w573 stop-if-true
            n420 = global read "Robot Global Data.vi" "Direction Commands"() -> (w582:T2)
            n421 = global read "Robot Global Data.vi" "Front Left Drive Position"() -> (w575:dbl)
            n422 = global read "Robot Global Data.vi" "Drive Commands"() -> (w581:T3)
            n423 = Bundle By Name(cluster=w582, "Lateral - X"=-0.3, "Longitudinal - Y"=0.0, "Rotational - Z"=0.0) -> (w588:T2)
            n424 = Bundle By Name(cluster=w581, "Align Steer Motors"=FALSE, "Brake"=FALSE, "Coast"=FALSE, "Autonomous"=TRUE) -> (w580:T3)
            n425 = global write "Robot Global Data.vi" "Reset Position"(FALSE ("Reset Position")) -> ()
            n426 = global write "Robot Global Data.vi" "Zero Yaw"(FALSE ("Zero Yaw")) -> ()
            n427 = global write "Robot Global Data.vi" "Direction Commands"(w588) -> ()
            n428 = global write "Robot Global Data.vi" "Align 90"(FALSE ("Auto Intake")) -> ()
            n429 = global write "Robot Global Data.vi" "Drive Commands"(w580) -> ()
            n430 = Absolute Value(x=w575) -> (abs(x)=w572:dbl)
            n431 = Greater Or Equal?(x=w572, y=12.0) -> (x >= y?=w573:bool)
          }
          n432 = global write "Robot Global Data.vi" "Auto Step"(2.0 ("Auto Step")) -> ()
          n433 = Wait (ms)(milliseconds to wait=u32 20) -> ()  [unwired: 1 out]
        }
        frame #10 {
          # "Align 90"
          n434 = global read "Robot Global Data.vi" "Direction Commands"() -> (w600:T2)
          n435 = global read "Robot Global Data.vi" "Drive Commands"() -> (w599:T3)
          n436 = global write "Robot Global Data.vi" "Auto Step"(4.0 ("Auto Step")) -> ()
          n437 = Bundle By Name(cluster=w600, "Lateral - X"=0.0, "Longitudinal - Y"=0.0, "Rotational - Z"=0.0) -> (w606:T2)
          n438 = Bundle By Name(cluster=w599, "Align Steer Motors"=FALSE, "Brake"=TRUE, "Coast"=FALSE, "Autonomous"=TRUE) -> (w598:T3)
          n439 = global write "Robot Global Data.vi" "Auto Shot left"(FALSE ("Auto Shot left")) -> ()
          n440 = global write "Robot Global Data.vi" "Reset Position"(TRUE ("Reset Position")) -> ()
          n441 = global write "Robot Global Data.vi" "Zero Yaw"(TRUE ("Zero Yaw")) -> ()
          n442 = global write "Robot Global Data.vi" "Auto Shot Right"(FALSE ("Auto Shot Right")) -> ()
          n443 = global write "Robot Global Data.vi" "Align 90"(FALSE ("Auto Intake")) -> ()
          n444 = global write "Robot Global Data.vi" "Direction Commands"(w606) -> ()
          n445 = global write "Robot Global Data.vi" "Drive Commands"(w598) -> ()
          n446 = Wait (ms)(milliseconds to wait=u32 400) -> ()  [unwired: 1 out]
        }
        frame #11 {
          # "Move Forward 8.5"
          n447 = while {
            stop <- w611 stop-if-true
            n448 = global read "Robot Global Data.vi" "Direction Commands"() -> (w620:T2)
            n449 = global read "Robot Global Data.vi" "Front Left Drive Position"() -> (w613:dbl)
            n450 = global read "Robot Global Data.vi" "Drive Commands"() -> (w619:T3)
            n451 = Bundle By Name(cluster=w620, "Lateral - X"=0.0, "Longitudinal - Y"=-0.2, "Rotational - Z"=0.0) -> (w626:T2)
            n452 = Bundle By Name(cluster=w619, "Align Steer Motors"=FALSE, "Brake"=FALSE, "Coast"=FALSE, "Autonomous"=TRUE) -> (w618:T3)
            n453 = global write "Robot Global Data.vi" "Reset Position"(FALSE ("Reset Position")) -> ()
            n454 = global write "Robot Global Data.vi" "Zero Yaw"(FALSE ("Zero Yaw")) -> ()
            n455 = global write "Robot Global Data.vi" "Direction Commands"(w626) -> ()
            n456 = global write "Robot Global Data.vi" "Align 90"(FALSE ("Auto Intake")) -> ()
            n457 = global write "Robot Global Data.vi" "Drive Commands"(w618) -> ()
            n458 = Absolute Value(x=w613) -> (abs(x)=w610:dbl)
            n459 = Greater Or Equal?(x=w610, y=8.5) -> (x >= y?=w611:bool)
          }
          n460 = global write "Robot Global Data.vi" "Auto Step"(2.0 ("Auto Step")) -> ()
          n461 = Wait (ms)(milliseconds to wait=u32 20) -> ()  [unwired: 1 out]
        }
        frame #12 {
          # "Wait"
          n462 = global read "Robot Global Data.vi" "Direction Commands"() -> (w638:T2)
          n463 = global read "Robot Global Data.vi" "Drive Commands"() -> (w637:T3)
          n464 = global write "Robot Global Data.vi" "Auto Step"(4.0 ("Auto Step")) -> ()
          n465 = Bundle By Name(cluster=w638, "Lateral - X"=0.0, "Longitudinal - Y"=0.0, "Rotational - Z"=0.0) -> (w644:T2)
          n466 = Bundle By Name(cluster=w637, "Align Steer Motors"=FALSE, "Brake"=TRUE, "Coast"=FALSE, "Autonomous"=TRUE) -> (w636:T3)
          n467 = global write "Robot Global Data.vi" "Auto Shot left"(FALSE ("Auto Shot left")) -> ()
          n468 = global write "Robot Global Data.vi" "Reset Position"(TRUE ("Reset Position")) -> ()
          n469 = global write "Robot Global Data.vi" "Zero Yaw"(TRUE ("Zero Yaw")) -> ()
          n470 = global write "Robot Global Data.vi" "Auto Shot Right"(FALSE ("Auto Shot Right")) -> ()
          n471 = global write "Robot Global Data.vi" "Align 90"(FALSE ("Auto Intake")) -> ()
          n472 = global write "Robot Global Data.vi" "Direction Commands"(w644) -> ()
          n473 = global write "Robot Global Data.vi" "Drive Commands"(w636) -> ()
          n474 = Wait (ms)(milliseconds to wait=u32 1200) -> ()  [unwired: 1 out]
        }
        frame #13 {
          # "Shoot Ball"
          n475 = global read "Robot Global Data.vi" "Direction Commands"() -> (w656:T2)
          n476 = global read "Robot Global Data.vi" "Drive Commands"() -> (w655:T3)
          n477 = global write "Robot Global Data.vi" "Auto Step"(4.0 ("Auto Step")) -> ()
          n478 = Bundle By Name(cluster=w656, "Lateral - X"=0.0, "Longitudinal - Y"=0.0, "Rotational - Z"=0.0) -> (w662:T2)
          n479 = Bundle By Name(cluster=w655, "Align Steer Motors"=TRUE, "Brake"=TRUE, "Coast"=FALSE, "Autonomous"=TRUE) -> (w654:T3)
          n480 = global write "Robot Global Data.vi" "Auto Shot left"(TRUE ("Auto Shot left")) -> ()
          n481 = global write "Robot Global Data.vi" "Reset Position"(TRUE ("Reset Position")) -> ()
          n482 = global write "Robot Global Data.vi" "Zero Yaw"(TRUE ("Zero Yaw")) -> ()
          n483 = global write "Robot Global Data.vi" "Auto Shot Right"(TRUE ("Auto Shot Right")) -> ()
          n484 = global write "Robot Global Data.vi" "Align 90"(FALSE ("Auto Intake")) -> ()
          n485 = global write "Robot Global Data.vi" "Direction Commands"(w662) -> ()
          n486 = global write "Robot Global Data.vi" "Drive Commands"(w654) -> ()
          n487 = Wait (ms)(milliseconds to wait=u32 400) -> ()  [unwired: 1 out]
        }
        frame #14 {
          # "End State"
          n488 = global read "Robot Global Data.vi" "Direction Commands"() -> (w672:T2)
          n489 = global read "Robot Global Data.vi" "Drive Commands"() -> (w671:T3)
          n490 = Bundle By Name(cluster=w672, "Lateral - X"=0.0, "Longitudinal - Y"=0.0, "Rotational - Z"=0.0) -> (w678:T2)
          n491 = Bundle By Name(cluster=w671, "Align Steer Motors"=FALSE, "Brake"=FALSE, "Coast"=FALSE, "Autonomous"=TRUE) -> (w670:T3)
          n492 = global write "Robot Global Data.vi" "Reset Position"(FALSE ("Reset Position")) -> ()
          n493 = global write "Robot Global Data.vi" "Zero Yaw"(FALSE ("Zero Yaw")) -> ()
          n494 = global write "Robot Global Data.vi" "Align 90"(FALSE ("Auto Intake")) -> ()
          n495 = global write "Robot Global Data.vi" "Auto Step"(5.0 ("Auto Step")) -> ()
          n496 = global write "Robot Global Data.vi" "Direction Commands"(w678) -> ()
          n497 = global write "Robot Global Data.vi" "Drive Commands"(w670) -> ()
          n498 = Wait (ms)(milliseconds to wait=u32 100) -> ()  [unwired: 1 out]
        }
      }
    }
    frame "1BallHigh" {
      n499 = flat-sequence {
        frame #0 {
          # "Align 0"
          # "Start"
          n500 = global write "Robot Global Data.vi" "Auto Step"(1.0 ("Auto Step")) -> ()
          n501 = global read "Robot Global Data.vi" "Direction Commands"() -> (w691:T2)
          n502 = global read "Robot Global Data.vi" "Drive Commands"() -> (w690:T3)
          n503 = Bundle By Name(cluster=w691, "Lateral - X"=0.0, "Longitudinal - Y"=0.0, "Rotational - Z"=0.0) -> (w697:T2)
          n504 = Bundle By Name(cluster=w690, "Align Steer Motors"=FALSE, "Brake"=TRUE, "Coast"=FALSE, "Autonomous"=TRUE) -> (w689:T3)
          n505 = global write "Robot Global Data.vi" "Reset Position"(TRUE ("Reset Position")) -> ()
          n506 = global write "Robot Global Data.vi" "Zero Yaw"(TRUE ("Zero Yaw")) -> ()
          n507 = global write "Robot Global Data.vi" "Auto Intake"(TRUE ("Auto Intake")) -> ()
          n508 = global write "Robot Global Data.vi" "Align 90"(TRUE ("Auto Intake")) -> ()
          n509 = global write "Robot Global Data.vi" "Direction Commands"(w697) -> ()
          n510 = global write "Robot Global Data.vi" "Drive Commands"(w689) -> ()
          n511 = global write "Robot Global Data.vi" "Auto Shot left"(FALSE ("Auto Shot left")) -> ()
          n512 = global write "Robot Global Data.vi" "Auto Shot Right"(FALSE ("Auto Shot Right")) -> ()
          n513 = Wait (ms)(milliseconds to wait=u32 400) -> ()  [unwired: 1 out]
        }
        frame #1 {
          # "Move Right 8.6"
          n514 = while {
            stop <- w702 stop-if-true
            n515 = global read "Robot Global Data.vi" "Direction Commands"() -> (w711:T2)
            n516 = global read "Robot Global Data.vi" "Front Left Drive Position"() -> (w704:dbl)
            n517 = global read "Robot Global Data.vi" "Drive Commands"() -> (w710:T3)
            n518 = Bundle By Name(cluster=w711, "Lateral - X"=-0.3, "Longitudinal - Y"=0.0, "Rotational - Z"=0.0) -> (w717:T2)
            n519 = Bundle By Name(cluster=w710, "Align Steer Motors"=FALSE, "Brake"=FALSE, "Coast"=FALSE, "Autonomous"=TRUE) -> (w709:T3)
            n520 = global write "Robot Global Data.vi" "Reset Position"(FALSE ("Reset Position")) -> ()
            n521 = global write "Robot Global Data.vi" "Zero Yaw"(FALSE ("Zero Yaw")) -> ()
            n522 = global write "Robot Global Data.vi" "Direction Commands"(w717) -> ()
            n523 = global write "Robot Global Data.vi" "Align 90"(FALSE ("Auto Intake")) -> ()
            n524 = global write "Robot Global Data.vi" "Drive Commands"(w709) -> ()
            n525 = Absolute Value(x=w704) -> (abs(x)=w701:dbl)
            n526 = Greater Or Equal?(x=w701, y=8.6) -> (x >= y?=w702:bool)
          }
          n527 = global write "Robot Global Data.vi" "Auto Step"(2.0 ("Auto Step")) -> ()
          n528 = Wait (ms)(milliseconds to wait=u32 20) -> ()  [unwired: 1 out]
        }
        frame #2 {
          # "Align 0"
          n529 = global read "Robot Global Data.vi" "Direction Commands"() -> (w727:T2)
          n530 = global read "Robot Global Data.vi" "Drive Commands"() -> (w726:T3)
          n531 = Bundle By Name(cluster=w727, "Lateral - X"=0.0, "Longitudinal - Y"=0.0, "Rotational - Z"=0.0) -> (w733:T2)
          n532 = Bundle By Name(cluster=w726, "Align Steer Motors"=TRUE, "Brake"=FALSE, "Coast"=FALSE, "Autonomous"=TRUE) -> (w725:T3)
          n533 = global write "Robot Global Data.vi" "Reset Position"(TRUE ("Reset Position")) -> ()
          n534 = global write "Robot Global Data.vi" "Zero Yaw"(FALSE ("Zero Yaw")) -> ()
          n535 = global write "Robot Global Data.vi" "Align 90"(FALSE ("Auto Intake")) -> ()
          n536 = global write "Robot Global Data.vi" "Auto Step"(5.0 ("Auto Step")) -> ()
          n537 = global write "Robot Global Data.vi" "Direction Commands"(w733) -> ()
          n538 = global write "Robot Global Data.vi" "Drive Commands"(w725) -> ()
          n539 = Wait (ms)(milliseconds to wait=u32 300) -> ()  [unwired: 1 out]
        }
        frame #3 {
          # "Move Back 18.4"
          n540 = while {
            stop <- w738 stop-if-true
            n541 = global read "Robot Global Data.vi" "Direction Commands"() -> (w747:T2)
            n542 = global read "Robot Global Data.vi" "Front Left Drive Position"() -> (w740:dbl)
            n543 = global read "Robot Global Data.vi" "Drive Commands"() -> (w746:T3)
            n544 = Bundle By Name(cluster=w747, "Lateral - X"=0.0, "Longitudinal - Y"=0.3, "Rotational - Z"=0.0) -> (w753:T2)
            n545 = Bundle By Name(cluster=w746, "Align Steer Motors"=FALSE, "Brake"=FALSE, "Coast"=FALSE, "Autonomous"=TRUE) -> (w745:T3)
            n546 = global write "Robot Global Data.vi" "Reset Position"(FALSE ("Reset Position")) -> ()
            n547 = global write "Robot Global Data.vi" "Zero Yaw"(FALSE ("Zero Yaw")) -> ()
            n548 = global write "Robot Global Data.vi" "Direction Commands"(w753) -> ()
            n549 = global write "Robot Global Data.vi" "Align 90"(FALSE ("Auto Intake")) -> ()
            n550 = global write "Robot Global Data.vi" "Drive Commands"(w745) -> ()
            n551 = Absolute Value(x=w740) -> (abs(x)=w737:dbl)
            n552 = Greater Or Equal?(x=w737, y=18.4) -> (x >= y?=w738:bool)
          }
          n553 = global write "Robot Global Data.vi" "Auto Step"(2.0 ("Auto Step")) -> ()
          n554 = Wait (ms)(milliseconds to wait=u32 20) -> ()  [unwired: 1 out]
        }
        frame #4 {
          # "Wait"
          n555 = global read "Robot Global Data.vi" "Direction Commands"() -> (w766:T2)
          n556 = global read "Robot Global Data.vi" "Drive Commands"() -> (w765:T3)
          n557 = Bundle By Name(cluster=w766, "Lateral - X"=0.0, "Longitudinal - Y"=0.0, "Rotational - Z"=0.0) -> (w772:T2)
          n558 = Bundle By Name(cluster=w765, "Align Steer Motors"=TRUE, "Brake"=FALSE, "Coast"=FALSE, "Autonomous"=TRUE) -> (w764:T3)
          n559 = global write "Robot Global Data.vi" "Reset Position"(TRUE ("Reset Position")) -> ()
          n560 = global write "Robot Global Data.vi" "Zero Yaw"(FALSE ("Zero Yaw")) -> ()
          n561 = global write "Robot Global Data.vi" "Auto Shot left"(FALSE ("Auto Shot left")) -> ()
          n562 = global write "Robot Global Data.vi" "Auto Shot Right"(FALSE ("Auto Shot Right")) -> ()
          n563 = global write "Robot Global Data.vi" "Align 90"(FALSE ("Auto Intake")) -> ()
          n564 = global write "Robot Global Data.vi" "Auto Step"(5.0 ("Auto Step")) -> ()
          n565 = global write "Robot Global Data.vi" "Auto Intake"(TRUE ("Auto Intake")) -> ()
          n566 = global write "Robot Global Data.vi" "Direction Commands"(w772) -> ()
          n567 = global write "Robot Global Data.vi" "Drive Commands"(w764) -> ()
          n568 = Wait (ms)(milliseconds to wait=u32 400) -> ()  [unwired: 1 out]
        }
        frame #5 {
          # "Shoot"
          n569 = global read "Robot Global Data.vi" "Direction Commands"() -> (w785:T2)
          n570 = global read "Robot Global Data.vi" "Drive Commands"() -> (w784:T3)
          n571 = Bundle By Name(cluster=w785, "Lateral - X"=0.0, "Longitudinal - Y"=0.0, "Rotational - Z"=0.0) -> (w791:T2)
          n572 = Bundle By Name(cluster=w784, "Align Steer Motors"=TRUE, "Brake"=FALSE, "Coast"=FALSE, "Autonomous"=TRUE) -> (w783:T3)
          n573 = global write "Robot Global Data.vi" "Reset Position"(TRUE ("Reset Position")) -> ()
          n574 = global write "Robot Global Data.vi" "Zero Yaw"(FALSE ("Zero Yaw")) -> ()
          n575 = global write "Robot Global Data.vi" "Auto Shot left"(TRUE ("Auto Shot left")) -> ()
          n576 = global write "Robot Global Data.vi" "Align 90"(FALSE ("Auto Intake")) -> ()
          n577 = global write "Robot Global Data.vi" "Auto Shot Right"(TRUE ("Auto Shot Right")) -> ()
          n578 = global write "Robot Global Data.vi" "Auto Step"(5.0 ("Auto Step")) -> ()
          n579 = global write "Robot Global Data.vi" "Direction Commands"(w791) -> ()
          n580 = global write "Robot Global Data.vi" "Auto Intake"(TRUE ("Auto Intake")) -> ()
          n581 = global write "Robot Global Data.vi" "Drive Commands"(w783) -> ()
          n582 = Wait (ms)(milliseconds to wait=u32 400) -> ()  [unwired: 1 out]
        }
        frame #6 {
          # "Move Back 30"
          n583 = while {
            stop <- w796 stop-if-true
            n584 = global read "Robot Global Data.vi" "Direction Commands"() -> (w805:T2)
            n585 = global read "Robot Global Data.vi" "Front Left Drive Position"() -> (w798:dbl)
            n586 = global read "Robot Global Data.vi" "Drive Commands"() -> (w804:T3)
            n587 = Bundle By Name(cluster=w805, "Lateral - X"=0.0, "Longitudinal - Y"=0.3, "Rotational - Z"=0.0) -> (w811:T2)
            n588 = Bundle By Name(cluster=w804, "Align Steer Motors"=FALSE, "Brake"=FALSE, "Coast"=FALSE, "Autonomous"=TRUE) -> (w803:T3)
            n589 = global write "Robot Global Data.vi" "Reset Position"(FALSE ("Reset Position")) -> ()
            n590 = global write "Robot Global Data.vi" "Zero Yaw"(FALSE ("Zero Yaw")) -> ()
            n591 = global write "Robot Global Data.vi" "Direction Commands"(w811) -> ()
            n592 = global write "Robot Global Data.vi" "Align 90"(FALSE ("Auto Intake")) -> ()
            n593 = global write "Robot Global Data.vi" "Drive Commands"(w803) -> ()
            n594 = Absolute Value(x=w798) -> (abs(x)=w795:dbl)
            n595 = Greater Or Equal?(x=w795, y=30.0) -> (x >= y?=w796:bool)
          }
          n596 = global write "Robot Global Data.vi" "Auto Step"(2.0 ("Auto Step")) -> ()
          n597 = Wait (ms)(milliseconds to wait=u32 20) -> ()  [unwired: 1 out]
        }
        frame #7 {
          # "End State"
          n598 = global read "Robot Global Data.vi" "Direction Commands"() -> (w822:T2)
          n599 = global read "Robot Global Data.vi" "Drive Commands"() -> (w821:T3)
          n600 = global write "Robot Global Data.vi" "Auto Intake"(FALSE ("Auto Intake")) -> ()
          n601 = Bundle By Name(cluster=w822, "Lateral - X"=0.0, "Longitudinal - Y"=0.0, "Rotational - Z"=0.0) -> (w828:T2)
          n602 = Bundle By Name(cluster=w821, "Align Steer Motors"=FALSE, "Brake"=FALSE, "Coast"=FALSE, "Autonomous"=TRUE) -> (w820:T3)
          n603 = global write "Robot Global Data.vi" "Reset Position"(FALSE ("Reset Position")) -> ()
          n604 = global write "Robot Global Data.vi" "Zero Yaw"(FALSE ("Zero Yaw")) -> ()
          n605 = global write "Robot Global Data.vi" "Align 90"(FALSE ("Auto Intake")) -> ()
          n606 = global write "Robot Global Data.vi" "Auto Step"(5.0 ("Auto Step")) -> ()
          n607 = global write "Robot Global Data.vi" "Direction Commands"(w828) -> ()
          n608 = global write "Robot Global Data.vi" "Drive Commands"(w820) -> ()
          n609 = Wait (ms)(milliseconds to wait=u32 300) -> ()  [unwired: 1 out]
        }
      }
    }
    frame "Move" {
      n610 = flat-sequence {
        frame #0 {
          # "Align 0"
          # "Start"
          n611 = global write "Robot Global Data.vi" "Auto Step"(1.0 ("Auto Step")) -> ()
          n612 = global read "Robot Global Data.vi" "Direction Commands"() -> (w839:T2)
          n613 = global read "Robot Global Data.vi" "Drive Commands"() -> (w838:T3)
          n614 = Bundle By Name(cluster=w839, "Lateral - X"=0.0, "Longitudinal - Y"=0.0, "Rotational - Z"=0.0) -> (w845:T2)
          n615 = Bundle By Name(cluster=w838, "Align Steer Motors"=TRUE, "Brake"=TRUE, "Coast"=FALSE, "Autonomous"=TRUE) -> (w837:T3)
          n616 = global write "Robot Global Data.vi" "Reset Position"(TRUE ("Reset Position")) -> ()
          n617 = global write "Robot Global Data.vi" "Zero Yaw"(TRUE ("Zero Yaw")) -> ()
          n618 = global write "Robot Global Data.vi" "Auto Intake"(FALSE ("Auto Intake")) -> ()
          n619 = global write "Robot Global Data.vi" "Align 90"(FALSE ("Auto Intake")) -> ()
          n620 = global write "Robot Global Data.vi" "Direction Commands"(w845) -> ()
          n621 = global write "Robot Global Data.vi" "Drive Commands"(w837) -> ()
          n622 = Wait (ms)(milliseconds to wait=u32 400) -> ()  [unwired: 1 out]
        }
        frame #1 {
          # "Move Back 42"
          n623 = while {
            stop <- w850 stop-if-true
            n624 = global read "Robot Global Data.vi" "Direction Commands"() -> (w859:T2)
            n625 = global read "Robot Global Data.vi" "Front Left Drive Position"() -> (w852:dbl)
            n626 = global read "Robot Global Data.vi" "Drive Commands"() -> (w858:T3)
            n627 = Bundle By Name(cluster=w859, "Lateral - X"=0.0, "Longitudinal - Y"=0.3, "Rotational - Z"=0.0) -> (w865:T2)
            n628 = Bundle By Name(cluster=w858, "Align Steer Motors"=TRUE, "Brake"=FALSE, "Coast"=FALSE, "Autonomous"=TRUE) -> (w857:T3)
            n629 = global write "Robot Global Data.vi" "Reset Position"(FALSE ("Reset Position")) -> ()
            n630 = global write "Robot Global Data.vi" "Zero Yaw"(FALSE ("Zero Yaw")) -> ()
            n631 = global write "Robot Global Data.vi" "Direction Commands"(w865) -> ()
            n632 = global write "Robot Global Data.vi" "Align 90"(FALSE ("Auto Intake")) -> ()
            n633 = global write "Robot Global Data.vi" "Drive Commands"(w857) -> ()
            n634 = Absolute Value(x=w852) -> (abs(x)=w849:dbl)
            n635 = Greater Or Equal?(x=w849, y=42.0) -> (x >= y?=w850:bool)
          }
          n636 = global write "Robot Global Data.vi" "Auto Step"(2.0 ("Auto Step")) -> ()
          n637 = Wait (ms)(milliseconds to wait=u32 20) -> ()  [unwired: 1 out]
        }
        frame #2 {
          # "End State"
          n638 = global read "Robot Global Data.vi" "Direction Commands"() -> (w875:T2)
          n639 = global read "Robot Global Data.vi" "Drive Commands"() -> (w874:T3)
          n640 = Bundle By Name(cluster=w875, "Lateral - X"=0.0, "Longitudinal - Y"=0.0, "Rotational - Z"=0.0) -> (w881:T2)
          n641 = Bundle By Name(cluster=w874, "Align Steer Motors"=FALSE, "Brake"=FALSE, "Coast"=FALSE, "Autonomous"=TRUE) -> (w873:T3)
          n642 = global write "Robot Global Data.vi" "Reset Position"(FALSE ("Reset Position")) -> ()
          n643 = global write "Robot Global Data.vi" "Zero Yaw"(FALSE ("Zero Yaw")) -> ()
          n644 = global write "Robot Global Data.vi" "Align 90"(FALSE ("Auto Intake")) -> ()
          n645 = global write "Robot Global Data.vi" "Auto Step"(5.0 ("Auto Step")) -> ()
          n646 = global write "Robot Global Data.vi" "Direction Commands"(w881) -> ()
          n647 = global write "Robot Global Data.vi" "Drive Commands"(w873) -> ()
          n648 = Wait (ms)(milliseconds to wait=u32 300) -> ()  [unwired: 1 out]
        }
      }
    }
  }
  n649 = while {
    stop <- FALSE stop-if-true
    n650 = global read "Robot Global Data.vi" "Navx  Comp Yaw"() -> (→"Navx  Comp Yaw":dbl)
    n651 = global read "Robot Global Data.vi" "Front Left Drive Position"() -> (→"Front Left Drive Position":dbl)
    n652 = global read "Robot Global Data.vi" "Auto Step"() -> (→"Auto Step":dbl)
  }
